vi "Drive Begin.vi"   [LabVIEW 2013]
uses:
  <vilib>/Rock Robotics/SystemInterfaces/DIO/FPGA_DIOPWMChannel.ctl
  <vilib>/Rock Robotics/SystemInterfaces/DIO/FPGA_DIOChannel.ctl
  <vilib>/Rock Robotics/SystemInterfaces/Typedef/FPGA_TypedefDigitalModule.ctl
  <vilib>/Rock Robotics/WPI/Encoder/WPI_EncoderType.ctl
  <vilib>/Rock Robotics/WPI/Joystick/WPI_JoystickDeviceEnum.ctl
  <vilib>/Rock Robotics/WPI/RobotDrive/WPI_RobotDriveOpen4MotorWithJaguar.vi
  <vilib>/Rock Robotics/WPI/Counter/WPI_CounterDigitalInputToDigitalSource.vi
types:
  T1 = typedef "WPI_JoystickDeviceEnum.ctl" = enum16{"USB 1", "USB 2", "USB 3", "USB 4", "Kinect 1", "Kinect 2"}
  T2 = typedef "WPI_EncoderType.ctl" = enum16{"1x", "2x", "4x"}
  T3 = typedef "FPGA_DIOChannel.ctl" = enum8{"DIO 1", "DIO 2", "DIO 3", "DIO 4", "DIO 5", "DIO 6", "DIO 7", "DIO 8", "DIO 9", "DIO 10", "DIO 11", "DIO 12", "DIO 13", "DIO 14", "Invalid"}
  T4 = typedef "FPGA_TypedefDigitalModule.ctl" = enum16{"Digital Module 1", "Digital Module 2"}
  T5 = typedef "FPGA_DIOPWMChannel.ctl" = enum8{"PWM 1", "PWM 2", "PWM 3", "PWM 4", "PWM 5", "PWM 6", "PWM 7", "PWM 8", "PWM 9", "PWM 10", "Invalid"}
  T6 = typedef "WPI_JoystickDevRef.ctl" = cluster{"Device":T1}
  T7 = typedef "WPI_RobotDriveDevRef.ctl" = cluster{"DevStatus":errorcluster, "Motors[]":T8[], "Square Inputs":bool, "Max Output":dbl, "Isochronous":bool}
  T8 = typedef "WPI_MotorControlDeviceRef.ctl" = cluster{"DeviceStatus":errorcluster, "Type":enum16{"PWM", "CAN"}, "PWM":cluster{"Digital Module":T4, "PWM Channel":T5, "DeadBand":T9}, "CAN":cluster{"Device Number":u8, "Control Mode":T10, "Semaphore":T11, "Max Vout":dbl}, "Invert":bool, "TransformRef":T12, "InvTransformRef":T12}
  T9 = typedef "WPI_PWMDeadband.ctl" = cluster{"Name":string, "maxPositivePwm":i32, "minPositivePwm":i32, "centerPwm":i32, "maxNegativePwm":i32, "minNegativePwm":i32, "angularRange":u16}
  T10 = typedef "WPI_CANJaguar_ControlMode.ctl" = enum8{"Percent VBus", "Current", "Speed", "Position", "Voltage"}
  T11 = typedef "Semaphore RefNum" = refnum<k1>
  T12 = typedef "WPI_PWMTransform_ConPane.ctl" = refnum<vi>
  T13 = typedef "WPI_DigitalInputDevRef.ctl" = cluster{"DevStatus":errorcluster, "DIO Channel":T3, "Digital Module":T4}
  T14 = typedef "FPGA_CounterEncoderSourceConvertionLVSourceType.ctl" = cluster{"DevStatus":errorcluster, "AnalogTriggerMode?":bool, "DigitalMode":cluster{"Digital Module":T4, "DIO Channel":T15}, "AnalogTriggerMode":cluster{"AnalogTriggerIndex":T16, "OutputType":T17}}
  T15 = typedef "FPGA_DIODigitalSourceChannel.ctl" = enum8{"DIO 1", "DIO 2", "DIO 3", "DIO 4", "DIO 5", "DIO 6", "DIO 7", "DIO 8", "DIO 9", "DIO 10", "DIO 11", "DIO 12", "DIO 13", "DIO 14", "Disabled"}
  T16 = typedef "FPGA_AnalogTriggerIndex.ctl" = enum8{"Trig 0", "Trig 1", "Trig 2", "Trig 3", "Trig 4", "Trig 5", "Trig 6", "Trig 7", "Invalid"}
  T17 = typedef "FPGA_AnalogTriggerOutType.ctl" = enum16{"InWindow", "TriggerState", "Rising", "Falling"}
  T18 = typedef "WPI_EncoderDevRef.ctl" = cluster{"DevStatus":errorcluster, "EncoderIndex":T19, "CounterIndex":T20, "DistancePerCount":dbl, "Decoding Type":T2}
  T19 = typedef "FPGA_EncoderIdx.ctl" = enum8{"Enc 0", "Enc 1", "Enc 2", "Enc 3", "Invalid"}
  T20 = typedef "FPGA_CounterCtrSystemIndex.ctl" = enum8{"Ctr 0", "Ctr 1", "Ctr 2", "Ctr 3", "Ctr 4", "Ctr 5", "Ctr 6", "Ctr 7", "Invalid"}
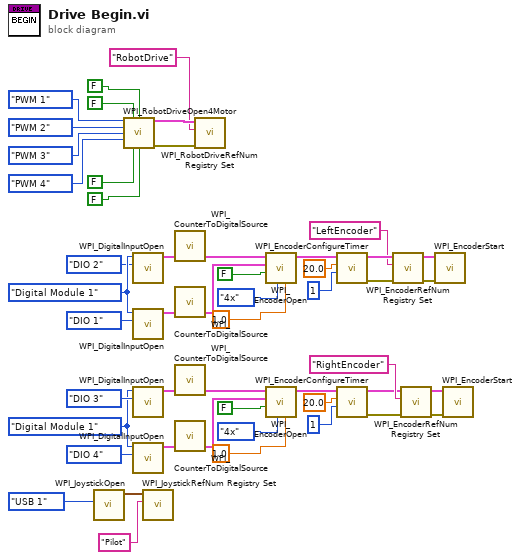
[diagram p0: block diagram]
diagram:
  w9 = FPGA_TypedefDigitalModule."Digital Module 1" ("Digital Module (Module 1)")
  w34 = FPGA_TypedefDigitalModule."Digital Module 1" ("Digital Module (Module 1)")
  n1 = call <vilib>:"WPI_JoystickOpen.vi"("JoystickDevice"=WPI_JoystickDeviceEnum."USB 1") -> ("JoystickDevRef"=w3:T6)  [unwired: 10 in]
  n2 = call-poly <vilib>:"WPI_RobotDriveOpen4Motor.vi"("Rear Left Motor"=FPGA_DIOPWMChannel."PWM 1", "Rear Left Motor Inverted"=FALSE, "Rear Right Motor Inverted"=FALSE, "Rear Right Motor"=FPGA_DIOPWMChannel."PWM 2", "Front Left Motor"=FPGA_DIOPWMChannel."PWM 3", "Front Right Motor"=FPGA_DIOPWMChannel."PWM 4", "Front Left Motor Inverted"=FALSE, "Front Right Motor Inverted"=FALSE) -> ("RobotDriveDevRef"=w42:T7, "error out"=w41:errorcluster)  [unwired: 6 in]
  n3 = call <vilib>:"WPI_DigitalInputOpen.vi"("DIO Channel"=FPGA_DIOChannel."DIO 2", "Digital Module (Module 1)"=w34) -> ("DigitalInputDevRef"=w37:T13)  [unwired: 1 in, 8 out]
  n4 = call <vilib>:"WPI_DigitalInputOpen.vi"("DIO Channel"=FPGA_DIOChannel."DIO 1", "Digital Module (Module 1)"=w34) -> ("DigitalInputDevRef"=w38:T13)  [unwired: 1 in, 8 out]
  n5 = call <vilib>:"WPI_DigitalInputOpen.vi"("DIO Channel"=FPGA_DIOChannel."DIO 3", "Digital Module (Module 1)"=w9) -> ("DigitalInputDevRef"=w5:T13)  [unwired: 1 in, 8 out]
  n6 = call <vilib>:"WPI_DigitalInputOpen.vi"("DIO Channel"=FPGA_DIOChannel."DIO 4", "Digital Module (Module 1)"=w9) -> ("DigitalInputDevRef"=w11:T13)  [unwired: 1 in, 8 out]
  n7 = call <vilib>:"WPI_JoystickRefNum Registry Set.vi"("refnum name"="Pilot", "JoystickDevRef"=w3) -> ()  [unwired: 8 in, 2 out]
  n8 = call-poly <vilib>:"WPI_CounterToDigitalSource.vi"("DigitalInputDevRef"=w37) -> ("Digital Source"=w36:T14)  [unwired: 6 out]
  n9 = call-poly <vilib>:"WPI_CounterToDigitalSource.vi"("DigitalInputDevRef"=w38) -> ("Digital Source"=w39:T14)  [unwired: 6 out]
  n10 = call-poly <vilib>:"WPI_CounterToDigitalSource.vi"("DigitalInputDevRef"=w5) -> ("Digital Source"=w4:T14)  [unwired: 6 out]
  n11 = call-poly <vilib>:"WPI_CounterToDigitalSource.vi"("DigitalInputDevRef"=w11) -> ("Digital Source"=w10:T14)  [unwired: 6 out]
  n12 = call <vilib>:"WPI_RobotDriveRefNum Registry Set.vi"("error in (no error)"=w41, "refnum name"="RobotDrive", "RobotDriveDevRef"=w42) -> ()  [unwired: 7 in, 2 out]
  n13 = call <vilib>:"WPI_EncoderOpen.vi"("DistancePerCount"=1.0, "Decoding Type"=WPI_EncoderType."4x", "Invert Direction (False)"=FALSE, "BSource"=w39, "ASource"=w36) -> ("EncoderDevRef"=w35:T18)  [unwired: 3 in, 3 out]
  n14 = call <vilib>:"WPI_EncoderOpen.vi"("DistancePerCount"=1.0, "Decoding Type"=WPI_EncoderType."4x", "Invert Direction (False)"=FALSE, "BSource"=w10, "ASource"=w4) -> ("EncoderDevRef"=w6:T18)  [unwired: 3 in, 3 out]
  n15 = call <vilib>:"WPI_EncoderConfigureTimer.vi"("Number Samples to Average"=u8 1, "Minimum Rate"=20.0, "EncoderDevRef"=w35) -> ("error out"=w24:errorcluster, "EncoderDevRef"=w26:T18)  [unwired: 1 in, 6 out]
  n16 = call <vilib>:"WPI_EncoderConfigureTimer.vi"("Number Samples to Average"=u8 1, "Minimum Rate"=20.0, "EncoderDevRef"=w6) -> ("error out"=w19:errorcluster, "EncoderDevRef"=w8:T18)  [unwired: 1 in, 6 out]
  n17 = call <vilib>:"WPI_EncoderRefNum Registry Set.vi"("error in (no error)"=w24, "refnum name"="LeftEncoder", "EncoderDevRef"=w26) -> ("error out"=w23:errorcluster, "EncoderDevRef"=w25:T18)  [unwired: 7 in]
  n18 = call <vilib>:"WPI_EncoderRefNum Registry Set.vi"("error in (no error)"=w19, "refnum name"="RightEncoder", "EncoderDevRef"=w8) -> ("error out"=w20:errorcluster, "EncoderDevRef"=w7:T18)  [unwired: 7 in]
  n19 = call <vilib>:"WPI_EncoderStart.vi"("error in (no error)"=w23, "EncoderDevRef"=w25) -> ()  [unwired: 10 out]
  n20 = call <vilib>:"WPI_EncoderStart.vi"("error in (no error)"=w20, "EncoderDevRef"=w7) -> ()  [unwired: 10 out]
